vi "WFGenA03PT.vi"(1 "Param 0: Frequency":dbl=2000.0, 2 "Param 1: Inactive":dbl, 3 "Param 2: Inactive":dbl, 4 "Param 3: Inactive":dbl, 5 "error in (no error)":errorcluster, 8 "WFParameters":T2={"Fs (Hz)"=100000.0, "Amp (V)"=5.0, "Ramp (s)"=0.005, "Dur (s)"=0.25} {"Dur (s)" min=0.0 format="%#_4g"; "Ramp (s)" min=0.0; "Fs (Hz)" min=0.0}, 10 "WFRepetitions":T1={"Del (s)"=0.0, "Int (s)"=0.0, "N"=1} {"Int (s)" min=0.0 format="%#_4g"; "Del (s)" min=0.0 format="%#_4f"}) -> (14 "Waveform Out":waveform(dbl)={"t0"=timestamp(0 s since 1904-01-01), "dt"=1e-05, "Y"=array[25000 elements]}, 19 "error out":errorcluster)   [LabVIEW 2013]
uses:
  WFParameters.ctl
  WFRepetitions.ctl
  util/impl/WFComposeA.vi
  <vilib>/measure/NI_MABase.lvlib
panel:
  out "Waveform Graph":waveform(dbl)(graph)={"t0"=timestamp(0 s since 1904-01-01), "dt"=1e-05, "Y"=array[25000 elements]}
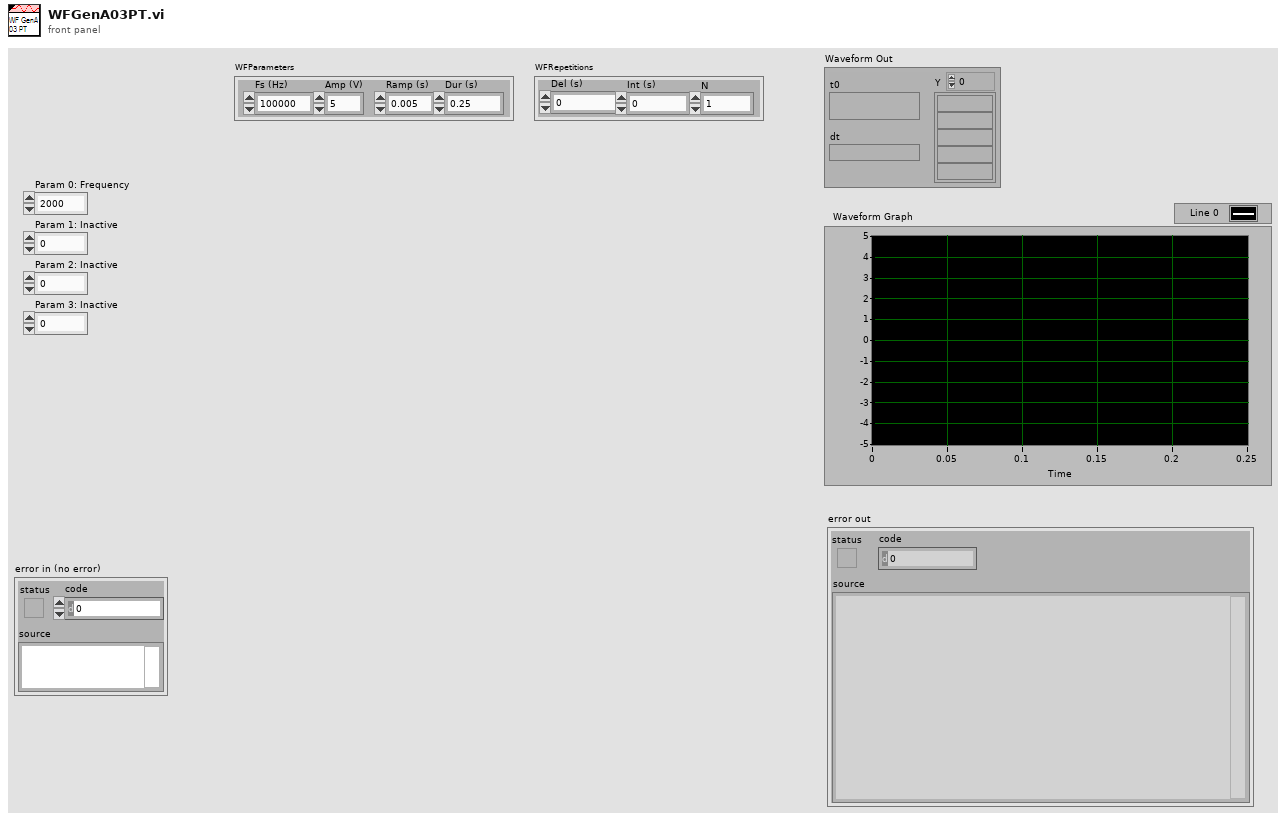
[diagram p1: front panel]
types:
  T1 = typedef "WFRepetitions.ctl" = cluster{"Del (s)":dbl, "Int (s)":dbl, "N":i32}
  T2 = typedef "WFParameters.ctl" = cluster{"Fs (Hz)":dbl, "Amp (V)":dbl, "Ramp (s)":dbl, "Dur (s)":dbl}
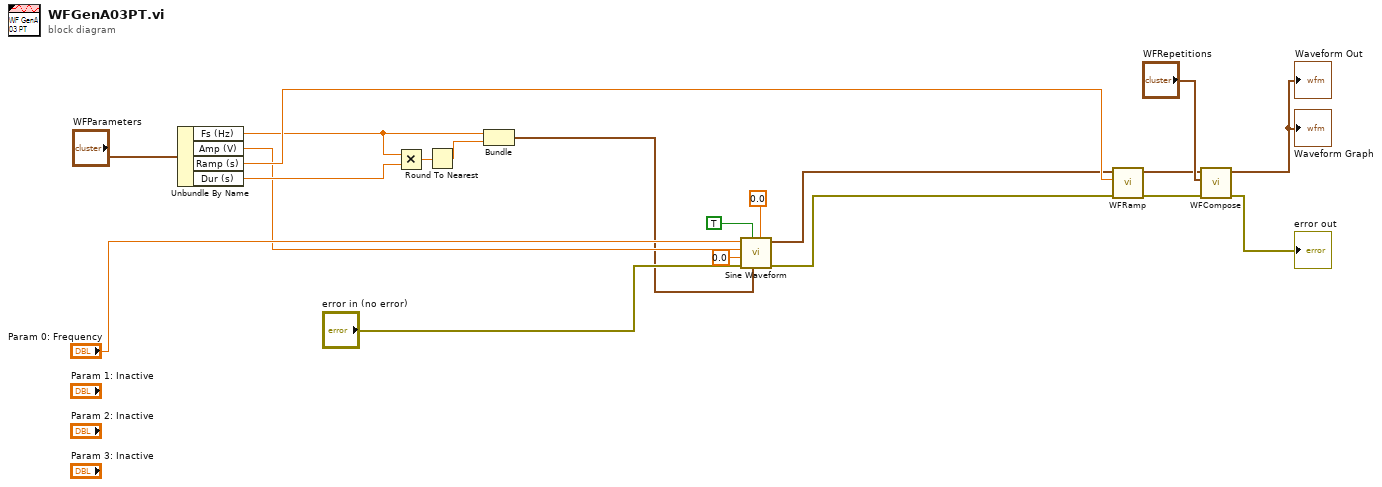
[diagram p0: block diagram]
diagram:
  n1 = Unbundle By Name("WFParameters") -> ("Fs (Hz)"=w4:dbl, "Amp (V)"=w9:dbl, "Ramp (s)"=w12:dbl, "Dur (s)"=w15:dbl)
  n2 = Multiply(x=w4, y=w15) -> (x*y=w16:dbl)
  n3 = Round To Nearest(number=w16) -> (nearest integer value=w3:dbl)
  n4 = Bundle("Fs (Hz)"=w4, w3) -> (w5:cluster{"Fs (Hz)":dbl, dbl})  [unwired: 1 in]
  n5 = call <vilib>:"Sine Waveform.vi"("offset"=0.0, "sampling info"=w5, "reset signal"=TRUE, "error in (no error)"="error in (no error)", "phase"=0.0, "amplitude"=w9, "frequency"="Param 0: Frequency") -> ("error out"=w2:errorcluster, "signal out"=w1:waveform(dbl))  [unwired: 3 in]
  n6 = call "WFRamp.vi"("error in (no error)"=w2, "Ramp Length (s)"=w12, "Waveform In"=w1) -> ("error out"=w13:errorcluster, "Waveform Out"=w14:waveform(dbl))  [unwired: 7 in]
  n7 = call-poly "WFCompose.vi"("error in (no error)"=w13, "WFRepetitions"="WFRepetitions", "Waveform In"=w14) -> ("error out"=→"error out":errorcluster, "Analog Waveform Out"=→"Waveform Graph" →"Waveform Out":waveform(dbl))  [unwired: 7 in]
